vi "Read_offsets_from_DB.vi"(9 "Assembly date":timestamp=timestamp(3857862657.9114094 s since 1904-01-01) format="%<%Y-%m-%d>T", 10 "Assembly Tray ID":string, 11 "Module?":bool) -> (1 "ang_offset_deg":dbl[](array[numeric]), 2 "y_offset_mm":dbl[](array[numeric]), 3 "x_offset_mm":dbl[](array[numeric]))   [LabVIEW 2021, in "Pick and Place.lvclass"]
uses:
  Pick and Place.lvclass
  <vilib>/Utility/file.llb/Read Delimited Spreadsheet (string).vi
panel:
  out "last mod":timestamp
  in  "No of modules requested":dbl
  out "No of returned entries":dbl
  out "Date text":string
  out "error out py":errorcluster
  in  "error in (no error) py":errorcluster
  out "DB offsets out":string[][](array[string])
  # "If no of modules requested is 0, it will return all modules"
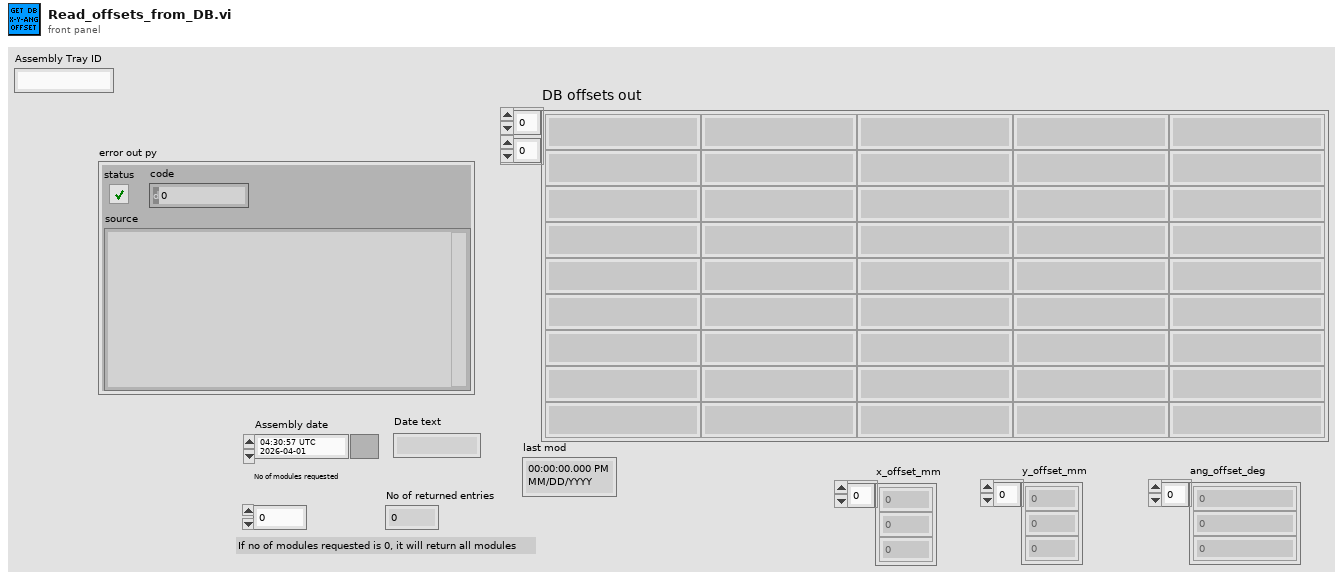
[diagram p1: front panel]
types:
  T1 = typedef "File Paths.ctl" = cluster{"Glue Pattern Folder":path, "Carrier Tray Folder":path, "Pick Up Tool Fixture Folder":path, "Components Folder":path, "Bellows Tool Offset.txt":path, "Pick Up Tool Offset.txt":path, "Dispense Tip Offset.txt":path, "Log Files":path, "Gantry Assembly Map.txt":path, "Syringe and offset map.txt":path, "Controllers Folder":path, "Local dbase config":path}
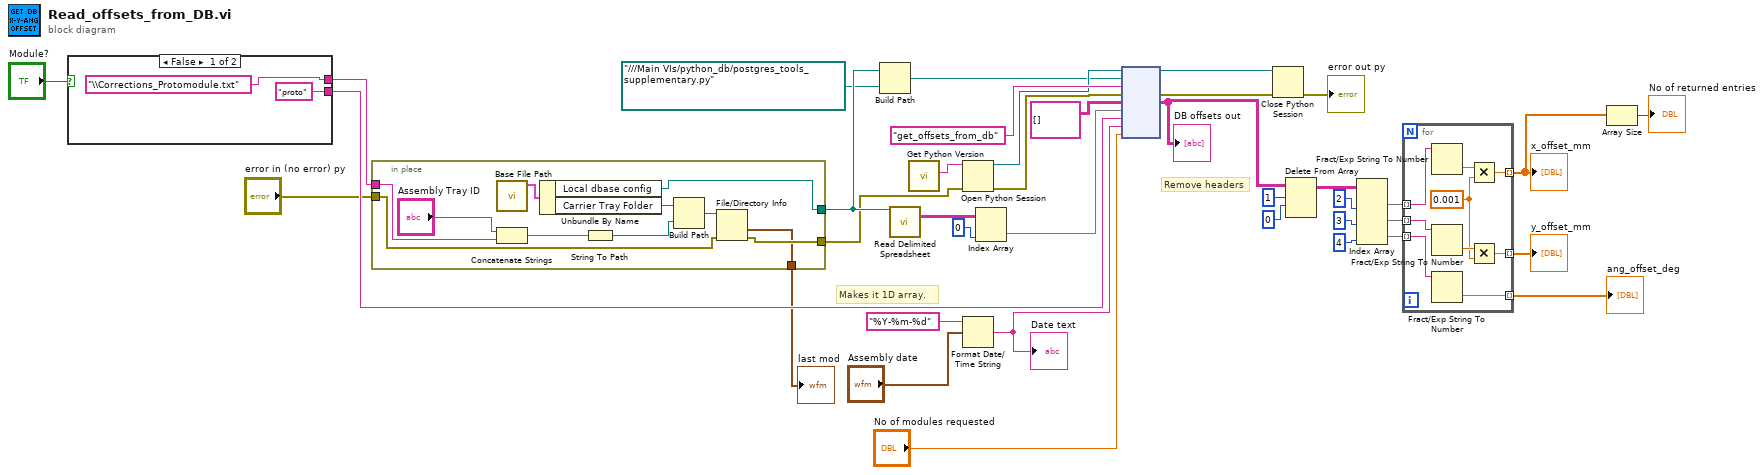
[diagram p0: block diagram]
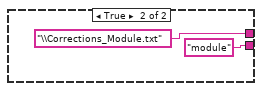
[diagram p2: hidden frame]
diagram:
  # "Remove headers"
  # "Makes it 1D array."
  n1 = case shown="False" "Module?" {
    tunnel: ["proto" "module"] -> w23
    tunnel: ["\\Corrections_Protomodule.txt" ("string") "\\Corrections_Module.txt" ("string")] -> w4
    frame False {
    }
    frame True {
    }
  }
  n2 = in-place {
    in-place-border: [w53] -> w36
    in-place-border: w4 -> [w49]
    in-place-border: "error in (no error) py" -> [w46]
    in-place-border: [w45] -> w2
    in-place-border: [w43] -> w1
    n3 = call "Base File Path.vi"() -> ("Paths Out"=w52:T1)  [unwired: 11 in]
    n4 = Concatenate Strings("Assembly Tray ID", w49) -> (w50:string)
    n5 = Unbundle By Name(w52) -> ("Local dbase config"=w53:path, "Carrier Tray Folder"=w51:path)
    n6 = String To Path(string=w50) -> (path=w48:path)
    n7 = Build Path(base path=w51, name or relative path=w48) -> (appended path=w47:path)
    n8 = File/Directory Info(path=w47, error in=w46) -> (last mod=w43:timestamp, error out=w45:errorcluster)  [unwired: 5 out]
  }
  "last mod" <- w1
  n9 = Build Path(base path=w36, name or relative path=path "../../../Main VIs/python_db/postgres_tools_supplementary.py" ("module path")) -> (appended path=w27:path)
  n10 = call-poly <vilib>:"Read Delimited Spreadsheet.vi"("file path (dialog if empty)"=w36) -> ("all rows"=w34:string[][])  [unwired: 9 in, 5 out]
  n11 = call "Get Python Version.vi"() -> ("Python Version"=w33:string)  [unwired: 10 in, 1 out]
  n12 = Open Python Session(python version=w33, 3:w2) -> (session out=w29:refnum<k35>, error out=w30:errorcluster)  [unwired: 1 in]
  n13 = Format Date/Time String(time format string (%c)="%Y-%m-%d", seconds (now)="Assembly date") -> (date/time string=w21:string)  [unwired: 1 in]
  "Date text" <- w21
  n14 = Index Array(array=w34, index (col)=0 ("disabled index (col)")) -> (element=w26:string[])  [unwired: 1 in]
  n15 = node(w29, w27, "get_offsets_from_db" ("function name"), w30, string[][] [], w26, w23, w21, "No of modules requested") -> (w25:refnum<k35>, w24:errorcluster, w17:string[][])  [unwired: 4 in, 2 out]
  "DB offsets out" <- w17
  n16 = Close Python Session(session in=w25, error in=w24) -> (11:→"error out py":errorcluster)
  n17 = Delete From Array(array=w17, length=1, index (row)=0) -> (array with subset deleted=w16:string[][])  [unwired: 1 in, 1 out]
  n18 = Index Array(array=w16, index (col) #1=2 ("index (row)"), index (col) #2=3 ("index (col)"), index (col) #3=4 ("index (col)")) -> (element #1=w15:string[], element #2=w12:string[], element #3=w9:string[])  [unwired: 3 in]
  n19 = for {
    tunnel: w15 -> [w62] mode=indexing
    tunnel: [w57] -> w7 mode=indexing
    tunnel: w12 -> [w61] mode=indexing
    tunnel: [w55] -> w11 mode=indexing
    tunnel: w9 -> [w60] mode=indexing
    tunnel: [w59] -> w8 mode=indexing
    w54 = 0.001 ("y")
    n20 = Fract/Exp String To Number(string=w62) -> (number=w58:dbl)  [unwired: 3 in, 1 out]
    n21 = Fract/Exp String To Number(string=w61) -> (number=w56:dbl)  [unwired: 3 in, 1 out]
    n22 = Fract/Exp String To Number(string=w60) -> (number=w59:dbl)  [unwired: 3 in, 1 out]
    n23 = Multiply(x=w58, y=w54) -> (x*y=w57:dbl)
    n24 = Multiply(x=w56, y=w54) -> (x*y=w55:dbl)
  }
  "x_offset_mm" <- w7
  "y_offset_mm" <- w11
  "ang_offset_deg" <- w8
  n25 = Array Size(array=w7) -> (size(s)=→"No of returned entries":i32)
